vi "Spectrometer Config.vi"() -> ()   [LabVIEW 2009, in "JY-SPEX-TRIAX.lvlib"]
uses:
  JY-SPEX-TRIAX.lvlib
  controls.llb/Monochromator System Number.ctl
panel:
  in  "Base Grating":dbl[unit]=1200000.0
  in  "Wavelength Backlash":dbl[unit]=1e-08
  in  "Slit Backlash":dbl[unit]=5e-05
  in  "Wavelength Min":dbl[unit]
  in  "Wavelength Max":dbl[unit]=1.4000000000000001e-06
  in  "Slit Min":dbl[unit]
  in  "Slit Max":dbl[unit]=0.0022400000000000002
  out "Mono System #":T1
  in  "Wavelength Step Rate":dbl[unit]=16000000000.0
  in  "Slit Step Rate":dbl[unit]=500000.0
  in  "Blaze Wavelength":dbl[unit][](array[numeric])=[5.000000000000001e-07, 7.5e-07, 1.0000000000000002e-06]
  in  "Groove Density":dbl[unit][](array[numeric])=[1200000.0, 1200000.0, 600000.0]
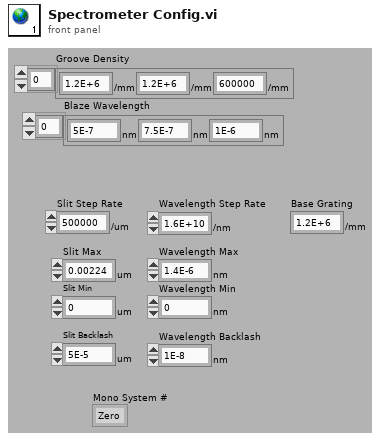
[diagram p1: front panel]
types:
  T1 = typedef "JY-SPEX-TRIAX.lvlib/Monochromator System Number.ctl" = enum16{"Zero", "One"}
diagram:
